vi "Error translator.vi"(8 "error in (no error)":errorcluster, 11 "error code":i32) -> (0 "error out":errorcluster)   [LabVIEW 2012]
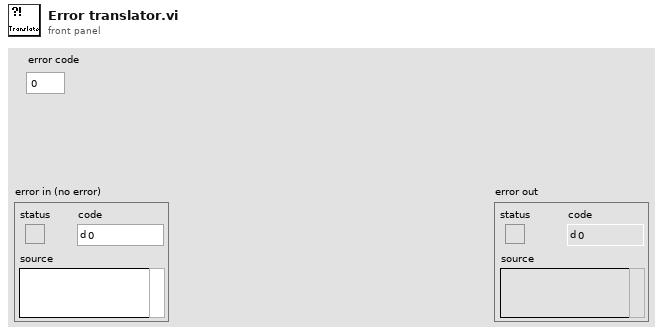
[diagram p1: front panel]
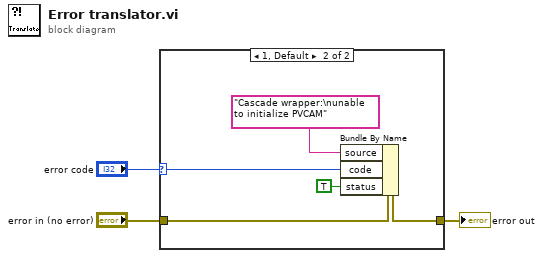
[diagram p0: block diagram]
diagram:
  n1 = case shown="1, Default" "error code" {
    selector: "error code" -> [_ w6]
    tunnel: [w4 w8] -> w2
    tunnel: "error in (no error)" -> [w4 w9]
    frame 0 {
    }
    frame 1, Default {
      n2 = Bundle By Name(cluster=w9, "source"="Cascade wrapper:\nunable to initialize PVCAM", "code"=w6, "status"=TRUE) -> (w8:errorcluster)
    }
  }
  "error out" <- w2
